vi "Filter_ChB(SubVI).vi"(10 "input":dbl, 11 "Filter on":bool) -> (2 "Output Number":dbl, 3 "Output":cluster{"Frequency Interpolate / Hz":dbl}(graph))   [LabVIEW 2015]
uses:
  <vilib>/ptbypt/NI_PtbyPt.lvlib
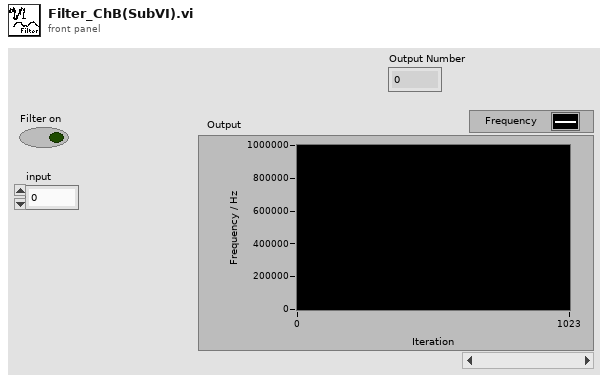
[diagram p1: front panel]
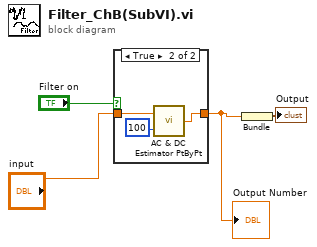
[diagram p0: block diagram]
diagram:
  n1 = case shown="True" "Filter on" {
    tunnel: "input" -> [w5 w7]
    tunnel: [w5 w6] -> w1
    frame False {
    }
    frame True {
      n2 = call <vilib>:"AC & DC Estimator PtByPt.vi"("signal"=w7, "sample length"=100) -> ("DC estimate (V)"=w6:dbl)  [unwired: 1 in, 2 out]
    }
  }
  "Output Number" <- w1
  n3 = Bundle("DC estimate (V)"=w1) -> (→"Output":cluster{"DC estimate (V)":dbl})  [unwired: 1 in]
